vi "Evaluate Transition Count.vi"(4 "Transition Count":u8) -> (2 "Idle?":bool)   [LabVIEW 2015]
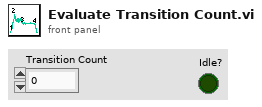
[diagram p1: front panel]
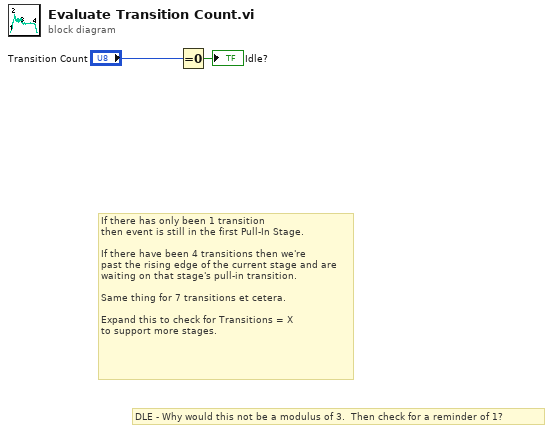
[diagram p0: block diagram]
diagram:
  # "DLE - Why would this not be a modulus of 3.  Then check for a reminder of 1?"
  # "If there has only been 1 transition\nthen event is still in the first Pull-In Stage.\n\nIf there have been 4 transitions then we're\npast the rising edge of the current stage and are\nwaiting on that stage's pull-in transition.\n\nSame thing for 7 transitions et cetera.\n\nExpand this to check for Transitions = X \nto support more stages."
  n1 = Equal To 0?(x="Transition Count") -> (x = 0?=→"Idle?":bool)
